vi "AlignCenter.vi"(6 "Variant in":variant, 7 "Shift Pressed?":bool, 8 "error in (no error)":errorcluster, 10 "QD Combo Box Ref":refnum<vi>, 11 "QD Launch VI Ref":refnum<vi>) -> (0 "error out":errorcluster, 4 "Variant out":variant)   [LabVIEW 2017]
doc: "Aligns center horizontally or vertically. To align vertically press Ctrl+Shift+c\n\nDefault Shortcut - [$c]"
panel:
  in  "Undo Name":string="Quick Drop Keyboard Shortcut"
  # "Do not change the connector pane of this VI.\n\nSee the block diagram for directions on how to use this template."
  # "Specify the name of the Undo transaction"
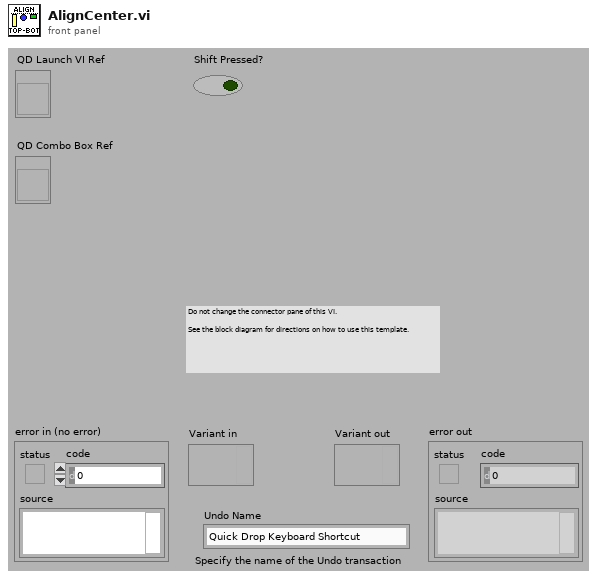
[diagram p1: front panel]
types:
  T1 = enum32{"Top Edges", "Vertical Centers", "Bottom Edges", "Left Edges", "Horizontal Centers", "Right Edges"}
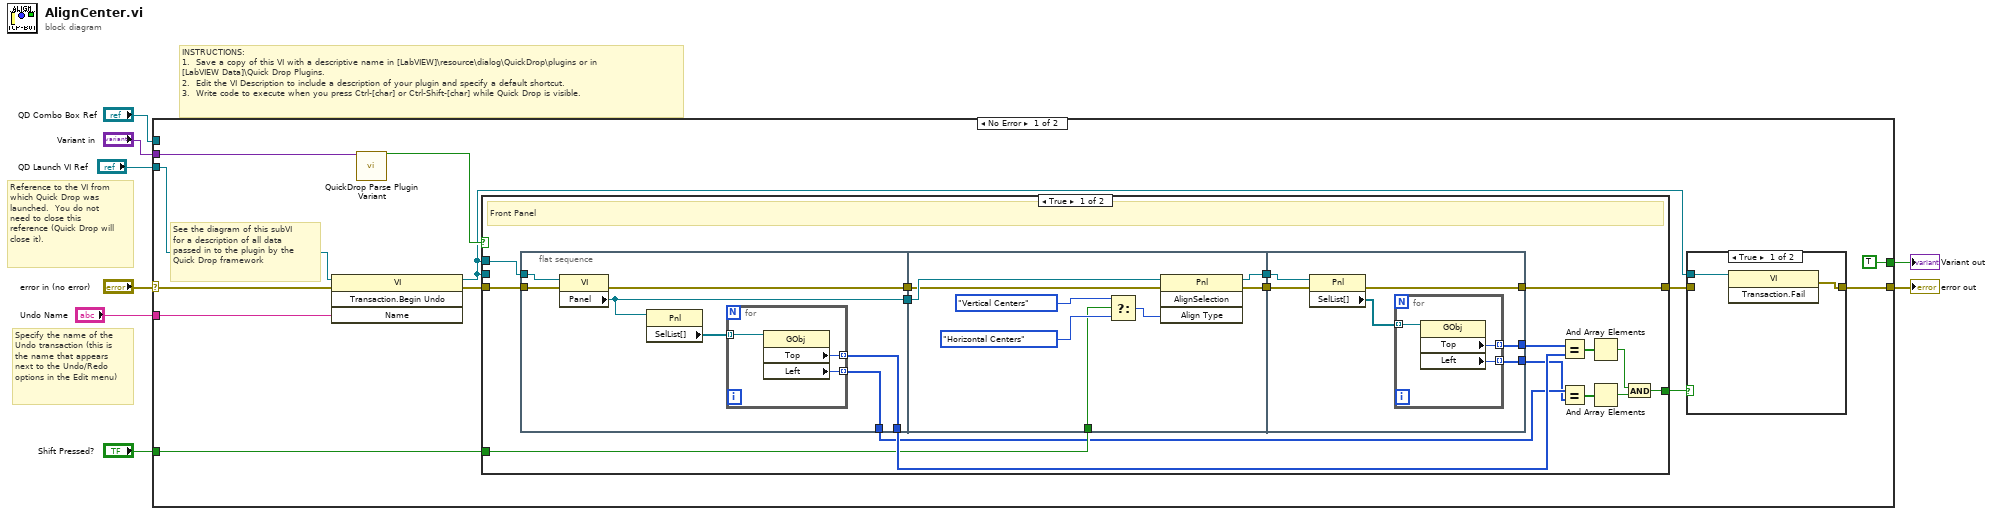
[diagram p0: block diagram]
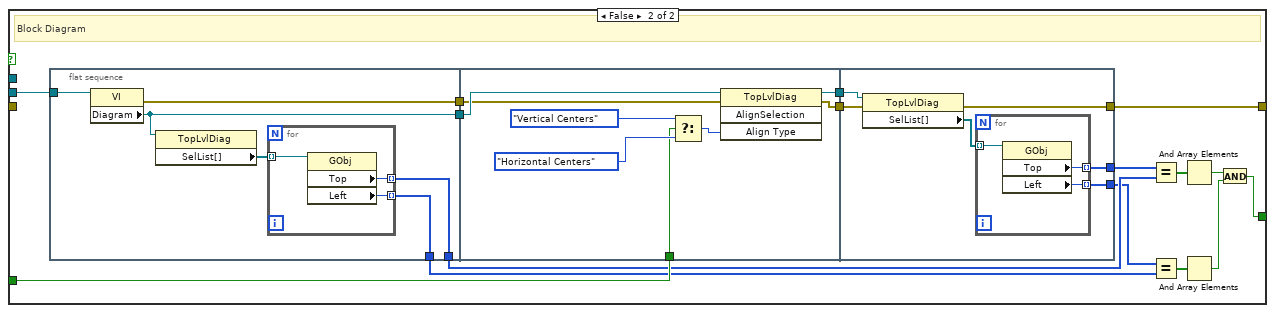
[diagram p2: hidden frame]
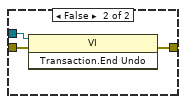
[diagram p3: hidden frame]
diagram:
  # "Specify the name of the Undo transaction (this is the name that appears next to the Undo/Redo options in the Edit menu)"
  # "Reference to the VI from which Quick Drop was launched.  You do not need to close this reference (Quick Drop will close it)."
  # "INSTRUCTIONS:\n1.  Save a copy of this VI with a descriptive name in [LabVIEW]\\resource\\dialog\\QuickDrop\\plugins or in [LabVIEW Data]\\Quick Drop Plugins.\n2.  Edit the VI Description to include a description of your plugin and specify a default shortcut. \n3.  Write code to execute when you press Ctrl-[char] or Ctrl-Shift-[char] while Quick Drop is visible."
  n1 = case shown="No Error" "error in (no error)" {
    selector: "error in (no error)" -> [w19 w112]
    tunnel: [w14 w112] -> w7
    tunnel: "QD Launch VI Ref" -> [w18 _]
    tunnel: "Shift Pressed?" -> [w11 _]
    tunnel: "QD Combo Box Ref" -> [_ _]
    tunnel: "Variant in" -> [w20 _]
    tunnel: "Undo Name" -> [w17 _]
    tunnel: [TRUE _] -> w1
    frame No Error {
      # "See the diagram of this subVI for a description of all data passed in to the plugin by the Quick Drop framework"
      n2 = invoke class="VI" method="Transaction.Begin Undo"(reference=w18, error in=w19, "Name"=w17) -> (reference out=w13:refnum<vi>, error out=w12:errorcluster)  [unwired: 1 in, 2 out]
      n3 = call <vilib>:"QuickDrop Parse Plugin Variant.vi"("QDKS Variant in"=w20) -> ("QD Launch VI Panel?"=w15:bool)  [unwired: 12 in, 2 out]
      n4 = case shown="True" w15 {
        tunnel: w12 -> [w29 _]
        tunnel: w13 -> [w30 _]
        tunnel: w13 -> [_ w80]
        tunnel: w11 -> [w26 w79]
        tunnel: [w27 w76] -> w10
        tunnel: [w24 w66] -> w9
        frame True {
          # "Front Panel"
          n5 = flat-sequence {
            tunnel: w30 -> [w44]
            tunnel: w29 -> [w43]
            tunnel: [w42] -> w37
            tunnel: [w41] -> w36
            tunnel: [w39] -> w32
            tunnel: [w38] -> w22
            tunnel: w37 -> [w52]
            tunnel: w36 -> [w51]
            tunnel: [w50] -> w35
            tunnel: [w49] -> w34
            tunnel: w26 -> [w48]
            tunnel: [w60] -> w27
            tunnel: w35 -> [w61]
            tunnel: w34 -> [w59]
            tunnel: [w57] -> w33
            tunnel: [w56] -> w21
            frame #0 {
              n6 = property class="VI"(reference=w44, error in=w43) -> (error out=w41:errorcluster, "Panel"=w42:refnum<vi>)  [unwired: 1 out]
              n7 = property class="Pnl"(reference=w42) -> ("SelList[]"=w40:refnum<vi>[])  [unwired: 1 in, 2 out]
              n8 = for {
                tunnel: [w47] -> w39 mode=indexing
                tunnel: w40 -> [w46] mode=indexing
                tunnel: [w45] -> w38 mode=indexing
                n9 = property class="GObj"(reference=w46) -> ("Top"=w47:i32, "Left"=w45:i32)  [unwired: 1 in, 2 out]
              }
            }
            frame #1 {
              n10 = Select(t=T1."Vertical Centers" ("Align Type"), s=w48, f=T1."Horizontal Centers" ("Align Type")) -> (s? t:f=w55:T1)
              n11 = invoke class="Pnl" method="AlignSelection"(reference=w52, error in=w51, "Align Type"=w55) -> (reference out=w49:refnum<vi>, error out=w50:errorcluster)  [unwired: 1 in, 2 out]
            }
            frame #2 {
              n12 = property class="Pnl"(reference=w59, error in=w61) -> (error out=w60:errorcluster, "SelList[]"=w58:refnum<vi>[])  [unwired: 1 out]
              n13 = for {
                tunnel: [w63] -> w57 mode=indexing
                tunnel: w58 -> [w64] mode=indexing
                tunnel: [w62] -> w56 mode=indexing
                n14 = property class="GObj"(reference=w64) -> ("Top"=w63:i32, "Left"=w62:i32)  [unwired: 1 in, 2 out]
              }
            }
          }
          n15 = Equal?(x=w33, y=w32) -> (x = y?=w31:bool[])
          n16 = Equal?(x=w22, y=w21) -> (x = y?=w25:bool[])
          n17 = And Array Elements(Boolean array=w31) -> (logical AND=w28:bool)
          n18 = And Array Elements(Boolean array=w25) -> (logical AND=w23:bool)
          n19 = And(x=w28, y=w23) -> (x .and. y?=w24:bool)
        }
        frame False {
          # "Block Diagram"
          n20 = flat-sequence {
            tunnel: w80 -> [w86]
            tunnel: [w85] -> w78
            tunnel: [w84] -> w77
            tunnel: [w82] -> w71
            tunnel: [w81] -> w68
            tunnel: w79 -> [w95]
            tunnel: w78 -> [w93]
            tunnel: w77 -> [w92]
            tunnel: [w91] -> w75
            tunnel: [w90] -> w74
            tunnel: [w102] -> w76
            tunnel: w75 -> [w103]
            tunnel: w74 -> [w101]
            tunnel: [w99] -> w72
            tunnel: [w98] -> w69
            frame #0 {
              n21 = property class="VI"(reference=w86) -> (error out=w84:errorcluster, "Diagram"=w85:refnum<vi>)  [unwired: 1 in, 1 out]
              n22 = property class="TopLvlDiag"(reference=w85) -> ("SelList[]"=w83:refnum<vi>[])  [unwired: 1 in, 2 out]
              n23 = for {
                tunnel: [w89] -> w82 mode=indexing
                tunnel: w83 -> [w88] mode=indexing
                tunnel: [w87] -> w81 mode=indexing
                n24 = property class="GObj"(reference=w88) -> ("Top"=w89:i32, "Left"=w87:i32)  [unwired: 1 in, 2 out]
              }
            }
            frame #1 {
              n25 = Select(t=T1."Vertical Centers" ("Align Type"), s=w95, f=T1."Horizontal Centers" ("Align Type")) -> (s? t:f=w97:T1)
              n26 = invoke class="TopLvlDiag" method="AlignSelection"(reference=w93, error in=w92, "Align Type"=w97) -> (reference out=w90:refnum<vi>, error out=w91:errorcluster)  [unwired: 1 in, 2 out]
            }
            frame #2 {
              n27 = property class="TopLvlDiag"(reference=w101, error in=w103) -> (error out=w102:errorcluster, "SelList[]"=w100:refnum<vi>[])  [unwired: 1 out]
              n28 = for {
                tunnel: [w105] -> w99 mode=indexing
                tunnel: w100 -> [w106] mode=indexing
                tunnel: [w104] -> w98 mode=indexing
                n29 = property class="GObj"(reference=w106) -> ("Top"=w105:i32, "Left"=w104:i32)  [unwired: 1 in, 2 out]
              }
            }
          }
          n30 = Equal?(x=w72, y=w71) -> (x = y?=w70:bool[])
          n31 = Equal?(x=w69, y=w68) -> (x = y?=w67:bool[])
          n32 = And Array Elements(Boolean array=w70) -> (logical AND=w73:bool)
          n33 = And Array Elements(Boolean array=w67) -> (logical AND=w65:bool)
          n34 = And(x=w73, y=w65) -> (x .and. y?=w66:bool)
        }
      }
      n35 = case shown="True" w9 {
        tunnel: w13 -> [w107 w110]
        tunnel: [w108 w111] -> w14
        tunnel: w10 -> [_ w109]
        frame True {
          n36 = invoke class="VI" method="Transaction.Fail"(reference=w107) -> (error out=w108:errorcluster)  [unwired: 2 in, 2 out]
        }
        frame False {
          n37 = invoke class="VI" method="Transaction.End Undo"(reference=w110, error in=w109) -> (error out=w111:errorcluster)  [unwired: 1 in, 2 out]
        }
      }
    }
    frame Error {
    }
  }
  "error out" <- w7
  "Variant out" <- w1
